vi "Scheduler-periodic.vi"(5 "Location, Network":u16(ring), 6 "Location, CL 2":u16(ring), 7 "Location, CL 1":u16(ring), 8 "Clock, plant 2":dbl, 9 "Region, plant 2":dbl, 10 "Clock, plant 1":dbl, 11 "Region, plant 1":dbl) -> (0 "Clock 2":i32, 1 "Clock 1":i32, 2 "Trigger?":bool, 3 "Plant to trigg":enum16{"Plant 1", "Plant 2"}(ring))   [LabVIEW 2016]
uses:
  <vilib>/Platform/TimedLoop/XDataNode/timing_clust.ctl
  <vilib>/Platform/TimedLoop/XDataNode/nitl_modes.ctl
  <vilib>/Platform/TimedLoop/XDataNode/wakeup.ctl
  <vilib>/Platform/TimedLoop/XDataNode/XDataNode.xnode
  <vilib>/Platform/TimedLoop/XDataNode/XDNodeRunTimeDep.lvlib
panel:
  in  "IET Plant 2":dbl(slide)=18.0 scale=10.0..50.0
  in  "IET Plant 1":dbl(slide)=28.0 scale=10.0..50.0
  # "The regions are provided by the plants/main loop;\nthe scheduler follows the UPPAAL-generated\nstrategy to decide the next steps to be taken"
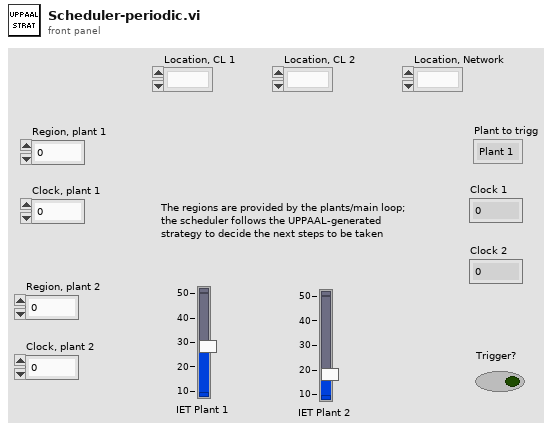
[diagram p1: front panel]
types:
  T1 = typedef "XDNodeRunTimeDep.lvlib/timing_clust.ctl" = cluster{"Expected End [f-1]":u64, "Actual End [f-1]":u64, "Finished Late? [f-1]":bool, "Expected End [i-1]":u64, "Actual End [i-1]":u64, "Finished Late? [i-1]":bool, "Expected Start [i]":u64, "Actual Start [i]":u64, "Expected Start [f]":u64, "Actual Start [f]":u64, "Source Name":string, "Structure Name":string, "Period":i64, "Deadline":i64, "Offset":i64, "Start":i64, "Priority":i32, "Timeout":i32, "Mode":T2, "Wakeup Reason":T3, "Error":errorcluster, "Source Type":string, "Secondary Source Type":string, "Global End Time":u64, "Global Start Time":u64, "Frame Duration":u64, "Iteration Duration":u64, "Assigned CPU":i32, "I/O Scan Engine Mode":u32}
  T2 = typedef "XDNodeRunTimeDep.lvlib/nitl_modes.ctl" = enum32{"No Change", "Process missed periods, maintain original phase", "Discard missed periods, maintain original phase", "Process missed periods, ignore original phase", "Discard missed periods, ignore original phase"}
  T3 = typedef "XDNodeRunTimeDep.lvlib/wakeup.ctl" = enum32{"Normal", "Aborted", "Asynchronous wakeup", "Timing source error", "Timed loop error", "Timeout"}
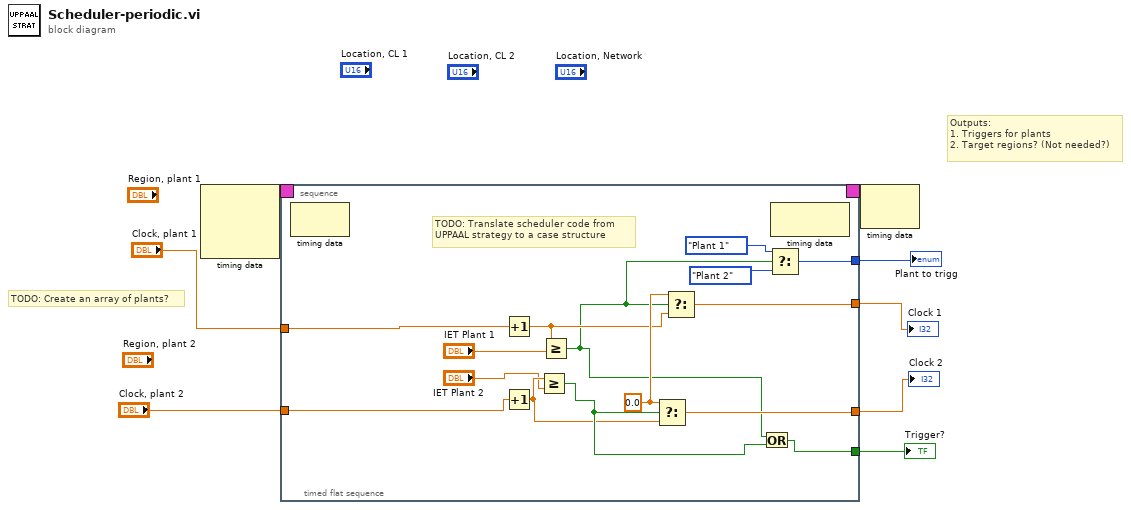
[diagram p0: block diagram]
diagram:
  # "Outputs:\n1. Triggers for plants\n2. Target regions? (Not needed?)"
  # "TODO: Create an array of plants?"
  n1 = node-c288() -> (w8:T1)  [unwired: 3 in]
  n2 = timed-sequence {
    timing: w8 -> [_]
    timing-out: [_] -> w7
    tunnel: "Clock, plant 1" -> [w14]
    tunnel: "Clock, plant 2" -> [w13]
    tunnel: [w12] -> w4
    tunnel: [w11] -> w3
    tunnel: [w10] -> w2
    tunnel: [w9] -> w1
    n3 = timed-flat-sequence {
      tunnel: w14 -> [w29]
      tunnel: w13 -> [w28]
      tunnel: [w26] -> w12
      tunnel: [w25] -> w11
      tunnel: [w22] -> w10
      tunnel: [w20] -> w9
      w24 = 0.0 ("t")
      # "TODO: Translate scheduler code from\nUPPAAL strategy to a case structure"
      n4 = node-c288() -> ()  [unwired: 1 in, 1 out]
      n5 = Increment(x=w29) -> (x+1=w23:dbl)
      n6 = Increment(x=w28) -> (x+1=w18:dbl)
      n7 = Greater Or Equal?(x=w18, y="IET Plant 2") -> (x >= y?=w19:bool)
      n8 = Greater Or Equal?(x=w23, y="IET Plant 1") -> (x >= y?=w21:bool)
      n9 = Select(t=w24, s=w19, f=w18) -> (s? t:f=w25:dbl)
      n10 = Select(t=w24, s=w21, f=w23) -> (s? t:f=w22:dbl)
      n11 = Or(x=w21, y=w19) -> (x .or. y?=w26:bool)
      n12 = Select(t=enum16{"Plant 1", "Plant 2"}."Plant 1" ("Plants"), s=w21, f=enum16{"Plant 1", "Plant 2"}."Plant 2" ("Plants")) -> (s? t:f=w20:enum16{"Plant 1", "Plant 2"})
      n13 = node-c288() -> ()  [unwired: 1 in, 1 out]
    }
  }
  "Clock 1" <- w2
  "Clock 2" <- w3
  "Trigger?" <- w4
  "Plant to trigg" <- w1
  n14 = node-c288(w7) -> ()  [unwired: 1 out]
